vi "Open.vi"(8 "error in (no error)":errorcluster, 11 "Serial in":refnum<class "Serial.lvclass">) -> (0 "error out":errorcluster, 3 "Serial out":refnum<class "Serial.lvclass">)   [LabVIEW 2018, in "Serial.lvclass"]
doc: "Serial.lvclass:Open.vi\n\nThis VI opens the serial port for communiication.\n\nInstrument Communication Module Version 1.0\nJuly, 2017 Original Code Consulting David Thomson\n www.originalcode.com"
uses:
  Serial.lvclass
  Serial.lvclass/Serial.ctl
  <vilib>/Instr/_visa.llb/VISA Configure Serial Port (Instr).vi
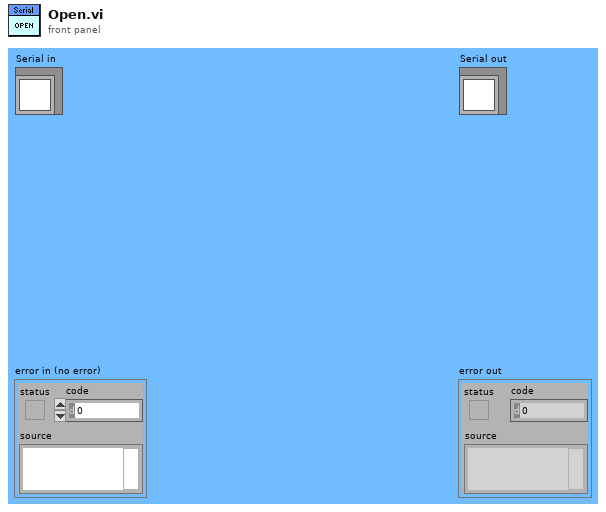
[diagram p1: front panel]
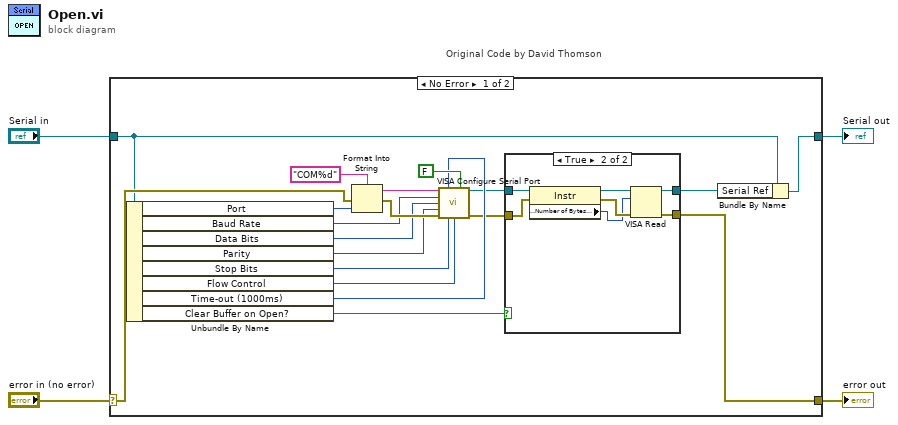
[diagram p0: block diagram]
diagram:
  n1 = case "Original Code by David Thomson" shown="No Error" "error in (no error)" {
    selector: "error in (no error)" -> [w21 w34]
    tunnel: [w7 w34] -> w3
    tunnel: [w5 w33] -> w1
    tunnel: "Serial in" -> [w6 w33]
    frame No Error {
      n2 = Unbundle By Name(w6) -> ("Port"=w23:i32, "Baud Rate"=w17:u32, "Data Bits"=w18:u16, "Parity"=w16:enum16{"None", "Odd", "Even", "Mark", "Space"}, "Stop Bits"=w15:u16, "Flow Control"=w13:u16, "Time-out (1000ms)"=w12:u32, "Clear Buffer on Open?"=w11:bool)
      n3 = Format Into String(format string="COM%d", error in=w21, w23) -> (resulting string=w20:string, error out=w19:errorcluster)  [unwired: 1 in]
      n4 = call-poly "VISA Configure Serial Port"("VISA resource name"=w20, "timeout (10sec)"=w12, "Enable Termination\nChar (T)"=FALSE ("Enable Termination\nChar (T)"), "baud rate (9600)"=w17, "data bits (8)"=w18, "parity (0:none)"=w16, "error in (no error)"=w19, "stop bits (10: 1 bit)"=w15, "flow control (0:none)"=w13) -> ("VISA resource name out"=w9:refnum<visa-resource-name>, "error out"=w10:errorcluster)  [unwired: 5 in]
      n5 = case shown="True" w11 {
        tunnel: w10 -> [w24 w32]
        tunnel: w9 -> [w25 w31]
        tunnel: [w24 w27] -> w7
        tunnel: [w25 w26] -> w8
        frame False {
        }
        frame True {
          n6 = property class="Instr"(reference=w31, error in=w32) -> (reference out=w30:refnum<visa-resource-name>, error out=w29:errorcluster, "Serial Settings:Number of Bytes at Serial Port"=w28:u32)
          n7 = VISA Read(VISA resource name=w30, byte count=w28, error in (no error)=w29) -> (VISA resource name out=w26:refnum<visa-resource-name>, error out=w27:errorcluster)  [unwired: 2 out]
        }
      }
      n8 = Bundle By Name(cluster=w6, "Serial Ref"=w8) -> (w5:refnum<class "Serial.lvclass">)
    }
    frame Error {
    }
  }
  "error out" <- w3
  "Serial out" <- w1
